vi "Special Data Types Example.vi"() -> ()   [LabVIEW 2024]
doc: "Minimal streaming example."
uses:
  Sift API/Types/Enum.ctl
  Sift API/Sift Client.lvclass
  Sift API/Types/Data Type.ctl
  Sift Client.lvlib
panel:
  out "URL":string
  in  "Run Name":string
  in  "Enum":T1
  out "Running":bool
  out "Flush Error":errorcluster
  in  "Stop":bool
  out "Error":errorcluster
  in  "API Key":string
  in  "API URL":string
  # "Special Data Types Example"
  # "Instructions\n\n1. Fill in the API URL, API Key, and Run Name. Visit this URL for more information on authentication\n    https://docs.siftstack.com/docs/api/authentication\n\n2. Start the VI\n\n3. Open the generated Run URL in a web browser to view the data. Plot the \"Enum Channel\" and \"String Channel\"."
  # "This example shows how to stream string and enum types.\n\nFill in the information below then open the corresponding Run in Sift\nto see data streaming in Live."
  # "Hit this to stop the example."
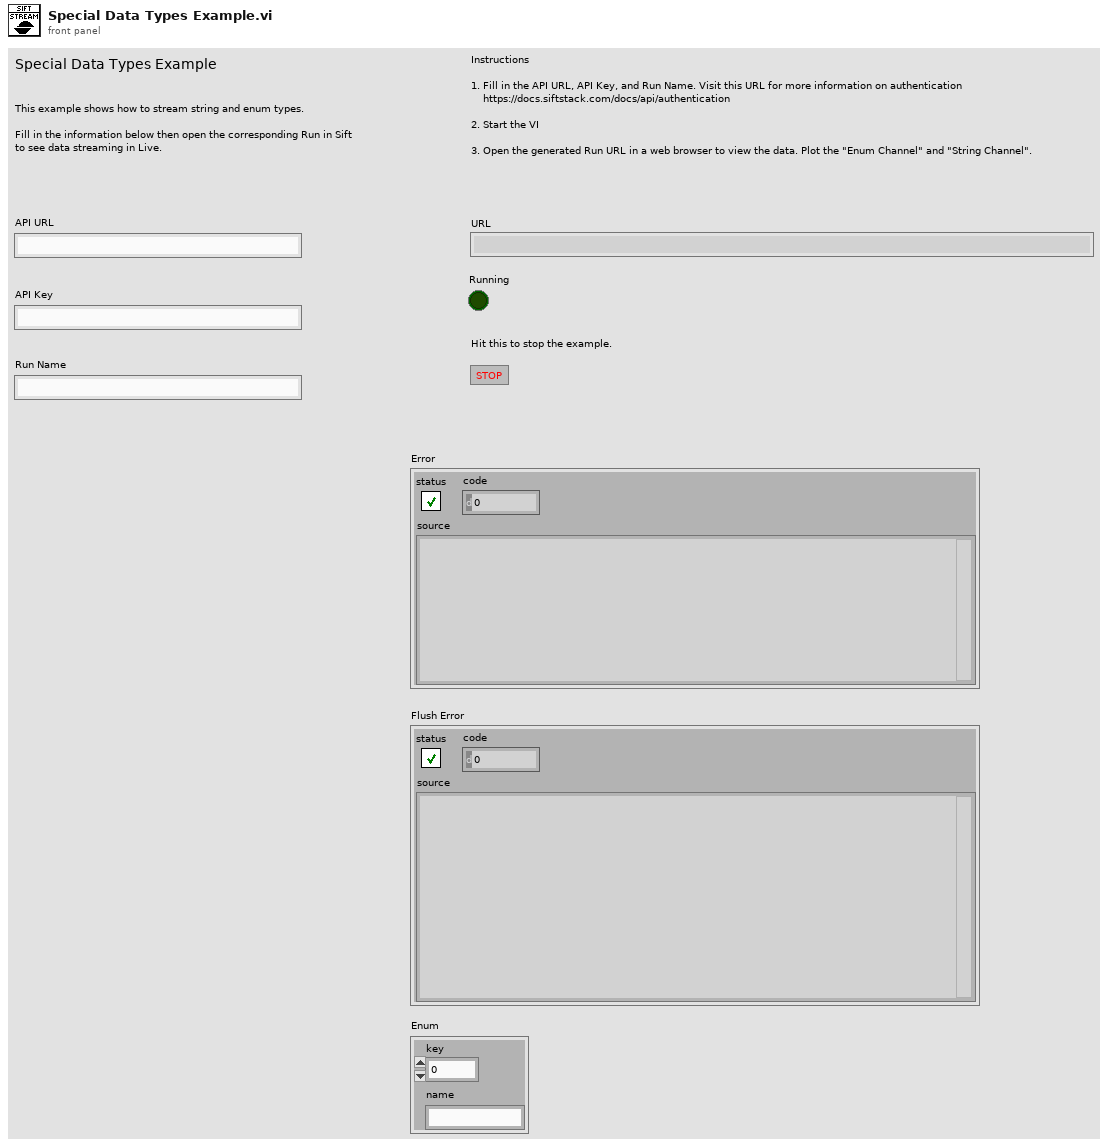
[diagram p1: front panel]
types:
  T1 = typedef "Sift Client.lvlib/Enum.ctl" = cluster{"key":u32, "name":string}
  T2 = typedef "Sift Client.lvlib/Data Type.ctl" = enum8{"double", "float", "uint64", "int64", "uint32", "int32", "bool", "enum", "string"}
  T3 = typedef "Sift Client.lvlib/Channel Config.ctl" = cluster{"name":string, "data_type":T2, "description":string, "component":string, "unit":string, "bit_field_elements":T4[], "enum_types":T1[]}
  T4 = typedef "Bit Field.ctl" = cluster{"index":u32, "bit_count":u32, "name":string}
  T5 = typedef "Sift Client.lvlib/Timestamp.ctl" = cluster{"seconds":i64, "nanos":i32}
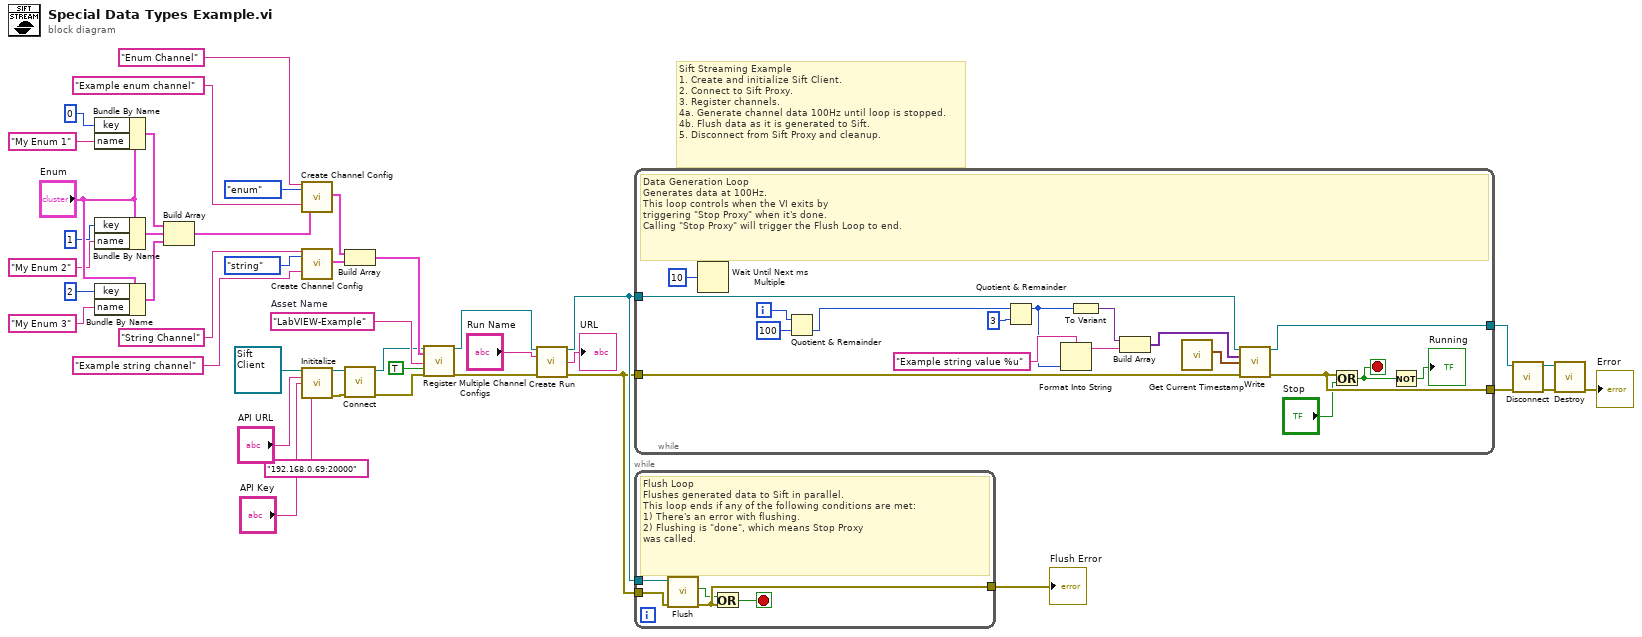
[diagram p0: block diagram]
diagram:
  w21 = "LabVIEW-Example"  # Asset Name
  # "Sift Streaming Example\n1. Create and initialize Sift Client.\n2. Connect to Sift Proxy.\n3. Register channels.\n4a. Generate channel data 100Hz until loop is stopped.\n4b. Flush data as it is generated to Sift.\n5. Disconnect from Sift Proxy and cleanup."
  n1 = Bundle By Name(cluster="Enum", "key"=u32 0 ("Key"), "name"="My Enum 1" ("Name")) -> (w17:T1)
  n2 = Bundle By Name(cluster="Enum", "key"=u32 1 ("Key"), "name"="My Enum 2" ("Name")) -> (w16:T1)
  n3 = Bundle By Name(cluster="Enum", "key"=u32 2 ("Key"), "name"="My Enum 3" ("Name")) -> (w15:T1)
  n4 = Build Array(w17, w16, w15) -> (w14:T1[])
  n5 = call "Create Channel Config.vi"("Name"="Enum Channel", "Data Type"=Data_Type."enum", "Description"="Example enum channel", "Enum Types"=w14) -> ("Output"=w25:T3)  [unwired: 15 in]
  n6 = call "Create Channel Config.vi"("Name"="String Channel", "Data Type"=Data_Type."string", "Description"="Example string channel") -> ("Output"=w24:T3)  [unwired: 16 in]
  n7 = call-dynamic "Inititalize.vi"("Sift Client in"=refnum<class "Sift Client.lvclass"> refnum ("Sift Client.lvlib:Sift Client.lvclass"), "API URL"="API URL", "API Key"="API Key", "Sift Proxy Address"="192.168.0.69:20000") -> ("Sift Client out"=w36:refnum<class "Sift Client.lvclass">, "error out"=w37:errorcluster)  [unwired: 10 in]
  n8 = Build Array(w25, w24) -> (w23:T3[])
  n9 = call-dynamic "Connect.vi"("error in (no error)"=w37, "Sift Client in"=w36) -> ("error out"=w22:errorcluster, "Sift Client out"=w19:refnum<class "Sift Client.lvclass">)  [unwired: 7 in, 1 out]
  n10 = call-dynamic "Register Multiple Channel Configs.vi"("Sift Client in"=w19, "Channel Configs"=w23, "Asset Name"=w21, "Submit Ingestion Config"=TRUE, "error in (no error)"=w22) -> ("Sift Client out"=w7:refnum<class "Sift Client.lvclass">, "error out"=w6:errorcluster)  [unwired: 12 in, 1 out]
  n11 = call-dynamic "Create Run.vi"("Sift Client in"=w7, "Name"="Run Name", "error in (no error)"=w6) -> ("Sift Client out"=w5:refnum<class "Sift Client.lvclass">, "URL"=→"URL":string, "error out"=w4:errorcluster)  [unwired: 9 in, 1 out]
  n12 = while {
    tunnel: w5 -> [w60]
    tunnel: w4 -> [w59]
    tunnel: [w54] -> w35
    tunnel: [w56] -> w34
    i -> [w47]
    stop <- w52 stop-if-true
    # "Data Generation Loop\nGenerates data at 100Hz.\nThis loop controls when the VI exits by \ntriggering \"Stop Proxy\" when it's done. \nCalling \"Stop Proxy\" will trigger the Flush Loop to end."
    n13 = Wait Until Next ms Multiple(millisecond multiple=u32 10 ("milliseconds to wait")) -> ()  [unwired: 1 out]
    n14 = Quotient & Remainder(x=w47, y=100) -> (floor(x/y)=w50:i32)  [unwired: 1 out]
    n15 = Quotient & Remainder(x=w50, y=3) -> (x-y*floor(x/y)=w44:i32)  [unwired: 1 out]
    n16 = Format Into String(format string="Example string value %u", w44) -> (resulting string=w43:string)  [unwired: 2 in, 1 out]
    n17 = To Variant(anything=w44) -> (Variant=w46:variant)
    n18 = Build Array(w46, w43) -> (w58:variant[])
    n19 = call "Get Current Timestamp.vi"() -> ("Timestamp"=w57:T5)  [unwired: 11 in]
    n20 = call-dynamic "Write.vi"("Sift Client in"=w60, "Values"=w58, "Timestamp"=w57, "error in (no error)"=w59) -> ("Sift Client out"=w54:refnum<class "Sift Client.lvclass">, "error out"=w56:errorcluster)  [unwired: 10 in]
    n21 = Or(x=w56, y="Stop") -> (x .or. y?=w52:bool)
    n22 = Not(x=w52) -> (.not. x?=→"Running":bool)
  }
  n23 = while {
    tunnel: w5 -> [w65]
    tunnel: [w63] -> w38
    tunnel: w4 -> [w64]
    stop <- w61 stop-if-true
    # "Flush Loop\nFlushes generated data to Sift in parallel.\nThis loop ends if any of the following conditions are met:\n1) There's an error with flushing.\n2) Flushing is \"done\", which means Stop Proxy \nwas called."
    n24 = call-dynamic "Flush.vi"("error in (no error)"=w64, "Sift Client in"=w65) -> ("error out"=w63:errorcluster, "Done"=w62:bool)  [unwired: 7 in, 1 out]
    n25 = Or(x=w62, y=w63) -> (x .or. y?=w61:bool)
  }
  "Flush Error" <- w38
  n26 = call-dynamic "Disconnect.vi"("error in (no error)"=w34, "Sift Client in"=w35) -> ("error out"=w33:errorcluster, "Sift Client out"=w32:refnum<class "Sift Client.lvclass">)  [unwired: 8 in]
  n27 = call-dynamic "Destroy.vi"("error in (no error)"=w33, "Sift Client in"=w32) -> ("error out"=→"Error":errorcluster)  [unwired: 8 in, 1 out]
